vi "Write Pre-Addressed Publish Message.vi"(10 "Pre-Addressed Publish Msg":refnum<class "Publish Msg.lvclass">, 11 "IModel in":refnum<class "IModel.lvclass">) -> (3 "IModel out":refnum<class "IModel.lvclass">)   [LabVIEW 2015, in "IModel.lvlib" / "IModel.lvclass"]
doc: "<License>\nCopyright © 2017 Composed Systems, LLC | All rights reserved\nwww.composed.io\n\nAuthor: Ethan Stern <ethan.stern@composed.io>\n\nThis software is provided \"AS IS\" WITHOUT WARRANTIES, either express or implied, AND IS FOR EDUCATIONAL PURPOSES ONLY.\n</License>"
uses:
  IModel.lvclass
  IMediator/IMediator Messages/Publish Msg/Publish Msg.lvclass
  IModel.lvclass/IModel.ctl
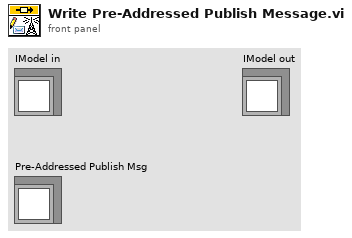
[diagram p1: front panel]
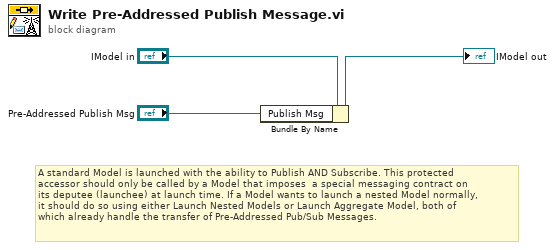
[diagram p0: block diagram]
diagram:
  # "A standard Model is launched with the ability to Publish AND Subscribe. This protected\naccessor should only be called by a Model that imposes  a special messaging contract on\nits deputee (launchee) at launch time. If a Model wants to launch a nested Model normally,\nit should do so using either Launch Nested Models or Launch Aggregate Model, both of\nwhich already handle the transfer of Pre-Addressed Pub/Sub Messages."
  n1 = Bundle By Name(cluster="IModel in", "Publish Msg"="Pre-Addressed Publish Msg") -> (→"IModel out":refnum<class "IModel.lvclass">)
